vi "OperationCycle.vi"(5 "EndTime":timestamp, 7 "StartTime":timestamp, 8 "error in":errorcluster, 11 "OperationRun":refnum<class "OperationCycle.lvclass">) -> (0 "error out":errorcluster, 3 "Passed":bool)   [LabVIEW 2020]
uses:
  <vilib>/Averna/ProligentResultProcessor/ProligentResultProcessor.lvlibp/OperationCycle/OperationCycle.lvclass
  <vilib>/Averna/ProligentResultProcessor/ProligentResultProcessor.lvlibp/OperationCycle/SetProcessFullName.vi
  <vilib>/Averna/ProligentResultProcessor/ProligentResultProcessor.lvlibp/OperationCycle/SetLocation.vi
  <vilib>/Averna/ProligentResultProcessor/ProligentResultProcessor.lvlibp/OperationCycle/SetOperationName.vi
  <vilib>/Averna/ProligentResultProcessor/ProligentResultProcessor.lvlibp/OperationCycle/SetOperationCycleStartTime.vi
  <vilib>/Averna/ProligentResultProcessor/ProligentResultProcessor.lvlibp/OperationCycle/SetUser.vi
  <vilib>/Averna/ProligentResultProcessor/ProligentResultProcessor.lvlibp/OperationCycle/SetOperationCycleStatus.vi
  <vilib>/Averna/ProligentResultProcessor/ProligentResultProcessor.lvlibp/OperationCycle/SetOperationCycleEndTime.vi
  <vilib>/Averna/ProligentResultProcessor/ProligentResultProcessor.lvlibp/OperationCycle/GetProcessFullName.vi
  <vilib>/Averna/ProligentResultProcessor/ProligentResultProcessor.lvlibp/OperationCycle/GetLocation.vi
  <vilib>/Averna/ProligentResultProcessor/ProligentResultProcessor.lvlibp/OperationCycle/GetOperationName.vi
  <vilib>/Averna/ProligentResultProcessor/ProligentResultProcessor.lvlibp/OperationCycle/GetOperationCycleStartTime.vi
  <vilib>/Averna/ProligentResultProcessor/ProligentResultProcessor.lvlibp/OperationCycle/GetUser.vi
  <vilib>/Averna/ProligentResultProcessor/ProligentResultProcessor.lvlibp/OperationCycle/GetOperationCycleStatus.vi
  <vilib>/Averna/ProligentResultProcessor/ProligentResultProcessor.lvlibp/OperationCycle/GetOperationCycleEndTime.vi
  <vilib>/Averna/ProligentResultProcessor/ProligentResultProcessor.lvlibp/OperationCycle/GetCustomData.vi
  <vilib>/Averna/ProligentResultProcessor/ProligentResultProcessor.lvlibp/Model/CustomData/CustomData.lvclass
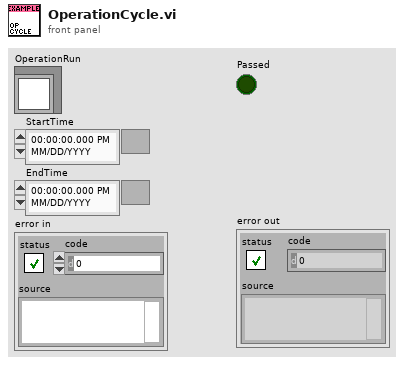
[diagram p1: front panel]
types:
  T1 = enum16{"PASS", "FAIL", "NOT_COMPLETED", "ABORTED"}
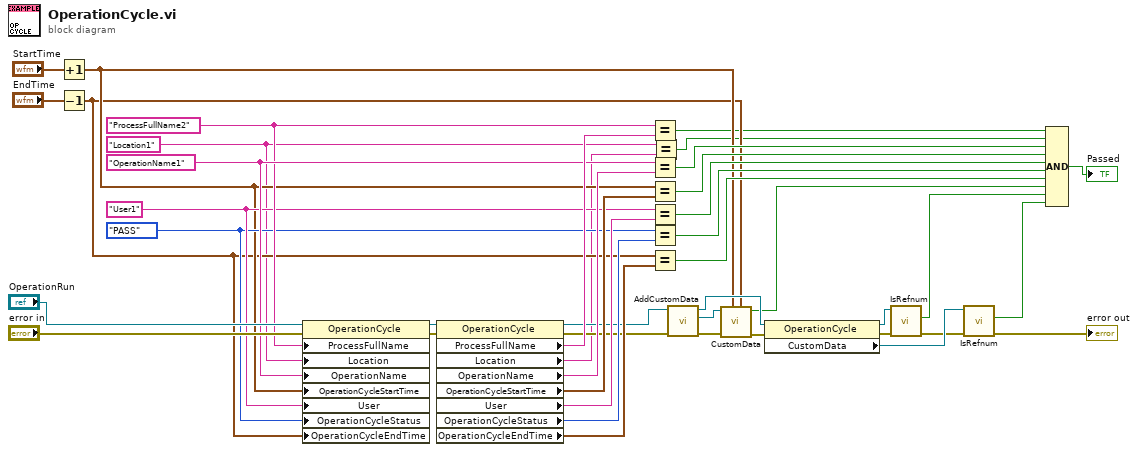
[diagram p0: block diagram]
diagram:
  w1 = "Location1"
  w22 = T1."PASS" ("ProcessRunStatus")
  w23 = "User1"
  w32 = "OperationName1"
  w31 = "ProcessFullName2"
  n1 = Increment(x="StartTime") -> (x+1=w11:timestamp)
  n2 = Decrement(x="EndTime") -> (x-1=w10:timestamp)
  n3 = property class="OperationCycle"(reference="OperationRun", error in="error in", "ProcessFullName"=w31, "Location"=w1, "OperationName"=w32, "OperationCycleStartTime"=w11, "User"=w23, "OperationCycleStatus"=w22, "OperationCycleEndTime"=w10) -> (reference out=w40:refnum<class "OperationCycle.lvclass">, error out=w39:errorcluster)
  n4 = property class="OperationCycle"(reference=w40, error in=w39) -> (reference out=w16:refnum<class "OperationCycle.lvclass">, error out=w17:errorcluster, "ProcessFullName"=w38:string, "Location"=w2:string, "OperationName"=w37:string, "OperationCycleStartTime"=w36:timestamp, "User"=w35:string, "OperationCycleStatus"=w34:T1, "OperationCycleEndTime"=w33:timestamp)
  n5 = Equal?(x=w31, y=w38) -> (x = y?=w4:bool)
  n6 = Equal?(x=w32, y=w37) -> (x = y?=w29:bool)
  n7 = Equal?(x=w11, y=w36) -> (x = y?=w28:bool)
  n8 = Equal?(x=w23, y=w35) -> (x = y?=w27:bool)
  n9 = Equal?(x=w22, y=w34) -> (x = y?=w26:bool)
  n10 = Equal?(x=w10, y=w33) -> (x = y?=w25:bool)
  n11 = Equal?(x=w1, y=w2) -> (x = y?=w3:bool)
  n12 = call <vilib>:"AddCustomData.vi"("error in"=w17, "Defect in"=w16) -> ("error out"=w15:errorcluster, "CustomData"=w14:refnum<class "CustomData.lvclass">, "Defect out"=w13:refnum<class "OperationCycle.lvclass">)  [unwired: 7 in]
  n13 = call "CustomData.vi"("EndTime"=w10, "StartTime"=w11, "error in"=w15, "CustomData"=w14) -> ("error out"=w12:errorcluster, "Passed"=w9:bool)  [unwired: 6 in]
  n14 = property class="OperationCycle"(reference=w13, error in=w12) -> (reference out=w19:refnum<class "OperationCycle.lvclass">, error out=w30:errorcluster, "CustomData"=w8:refnum<class "CustomData.lvclass">)
  n15 = call <vilib>:"IsRefnum.vi"("error in"=w30, "OperationCycle in"=w19) -> ("error out"=w7:errorcluster, "IsRefnum"=w18:bool)  [unwired: 7 in, 1 out]
  n16 = call <vilib>:"IsRefnum.vi"("error in"=w7, "CustomDataType in"=w8) -> ("error out"=→"error out":errorcluster, "IsRefnum"=w5:bool)  [unwired: 7 in, 1 out]
  n17 = Compound Arithmetic op=AND(w4, w3, w29, w28, w27, w26, w25, w9, w18, w5) -> (→"Passed":bool)
